vi "Switch Channel.vi"(8 "error in (no error)":errorcluster, 9 "CH2":string, 10 "CH1":string, 11 "PEU in":refnum<class "PEU.lvclass">) -> (0 "error out":errorcluster, 3 "PEU out":refnum<class "PEU.lvclass">)   [LabVIEW 2020, in "PEU.lvlib" / "PEU.lvclass"]
uses:
  PEU.lvclass
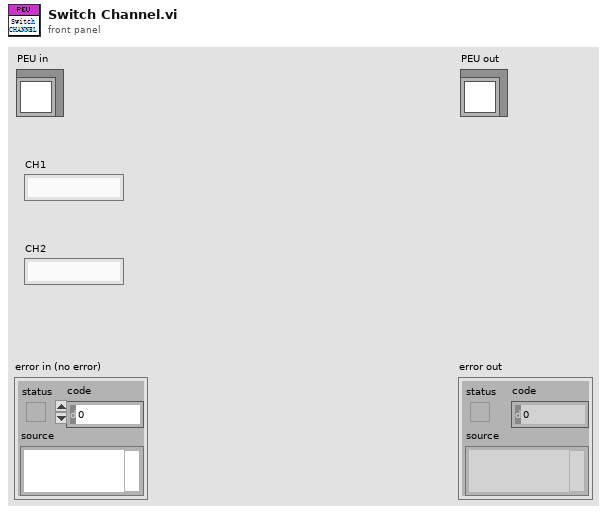
[diagram p1: front panel]
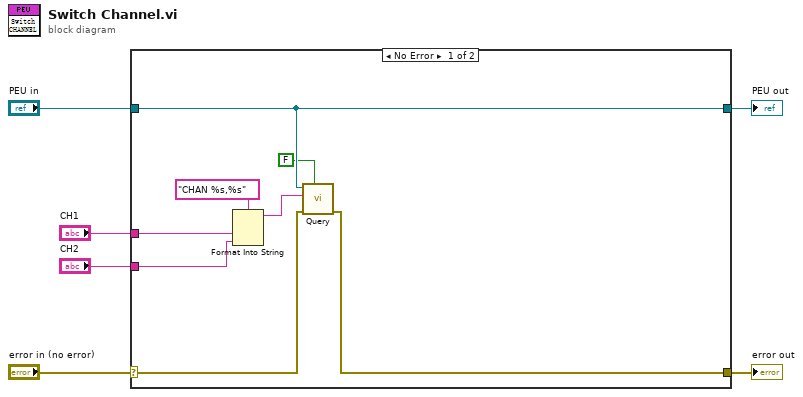
[diagram p0: block diagram]
diagram:
  n1 = case shown="No Error" "error in (no error)" {
    selector: "error in (no error)" -> [w12 w16]
    tunnel: [w11 w16] -> w5
    tunnel: [w14 w15] -> w3
    tunnel: "PEU in" -> [w14 w15]
    tunnel: "CH1" -> [w9 _]
    tunnel: "CH2" -> [w8 _]
    frame No Error {
      n2 = Format Into String(format string="CHAN %s,%s", w9, w8) -> (resulting string=w7:string)  [unwired: 2 in, 1 out]
      n3 = call "Query.vi"("Return"=FALSE, "error in (no error)"=w12, "Command"=w7, "PEU in"=w14) -> ("error out"=w11:errorcluster)  [unwired: 5 in, 2 out]
    }
    frame Error {
    }
  }
  "error out" <- w5
  "PEU out" <- w3
